vi "Register for Stimulus Profile Session Undeploy Event.vi"(8 "error in (no error)":errorcluster, 11 "Session Ref in":T2) -> (0 "error out":errorcluster, 2 "Event Registration Refnum":refnum<event-registration>, 3 "Session Ref out":T2, 5 "Session Undeploy Event Ref":T1)   [LabVIEW 2020, in "NI_VS Sequence Execution Interface.lvlib"]
doc: "Registers for a session undeploy event for the session you specify. A session undeploy event is triggered when the session undeploys from a target. This VI returns a registered user event reference and information about the event."
uses:
  <vilib>/NI VeriStand/Execution/SequenceExecutionInterface/NI_VS Sequence Execution Interface.lvlib
  <vilib>/NI VeriStand/Execution/SequenceExecutionInterface/Stimulus Profile Session Ref.ctl
  NationalInstruments.VeriStand.ClientAPI
  <vilib>/NI VeriStand/Execution/SequenceExecutionInterface/Session Event Ref.ctl
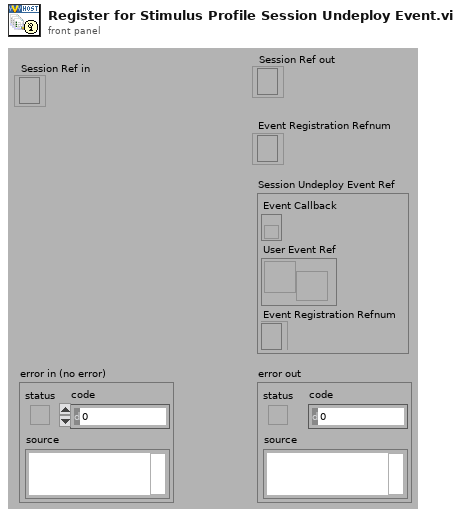
[diagram p1: front panel]
types:
  T1 = typedef "NI_VS Sequence Execution Interface.lvlib/Session Event Ref.ctl" = cluster{"Event Callback":refnum<k27>, "User Event Ref":refnum<user-event>, "Event Registration Refnum":refnum<event-registration>}
  T2 = typedef "NI_VS Sequence Execution Interface.lvlib/Stimulus Profile Session Ref.ctl" = refnum<k24>
  T3 = cluster{refnum<k27>, "Session Ref":refnum<user-event>, "Event Registration Refnum":refnum<event-registration>}
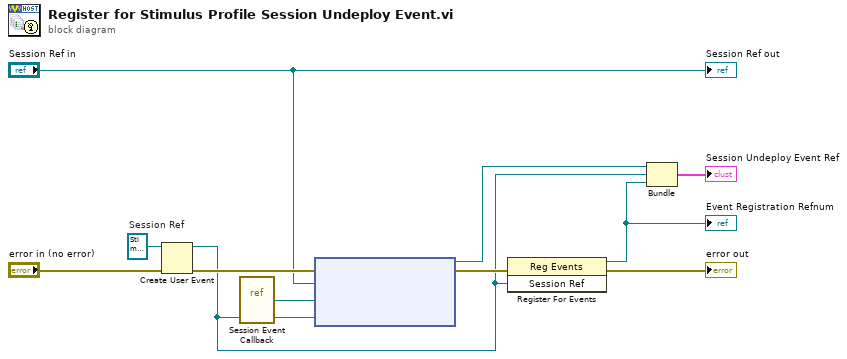
[diagram p0: block diagram]
diagram:
  w8 = T2 refnum  # Session Ref
  n1 = Create User Event(user event datatype=w8, error in="error in (no error)") -> (user event=w1:refnum<user-event>, error out=w11:errorcluster)
  n2 = vi-ref <vilib>:"Session Event Callback.vi"() -> ("vi reference"=w9:refnum<vi>)
  n3 = node(w11, "Session Ref in", w9, w1) -> (w6:refnum<k27>, w4:errorcluster)  [unwired: 1 in]
  n4 = register-events(error in=w4, w1) -> (reference out=w2:refnum<event-registration>, error out=→"error out":errorcluster)  [unwired: 1 in]
  "Event Registration Refnum" <- w2
  n5 = Bundle(w6, "Session Ref"=w1, "Event Registration Refnum"=w2) -> (→"Session Undeploy Event Ref":T3)  [unwired: 1 in]
  "Session Ref out" <- "Session Ref in"
